vi "Update Available Channels.vi"(8 "error in (no error)":errorcluster) -> (0 "error out":errorcluster)   [LabVIEW 2016]
uses:
  <vilib>/TagLibrary/Create Tag (String).vi
  <vilib>/TagLibrary/Write (String).vi
  <vilib>/TagLibrary/Tag Library.lvlib
  <resource>/objmgr/daqmx.rc
  <vilib>/TagLibrary/Close Tag (Single).vi
panel:
  out "System Tag":string
  out "JSON string":string
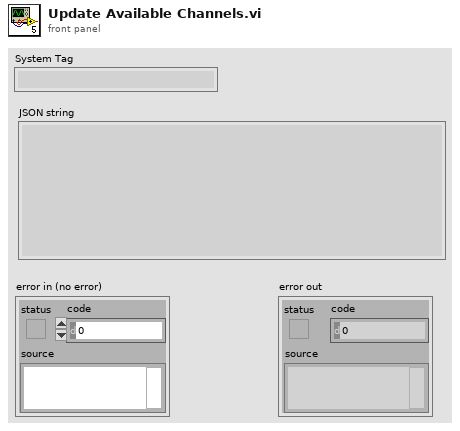
[diagram p1: front panel]
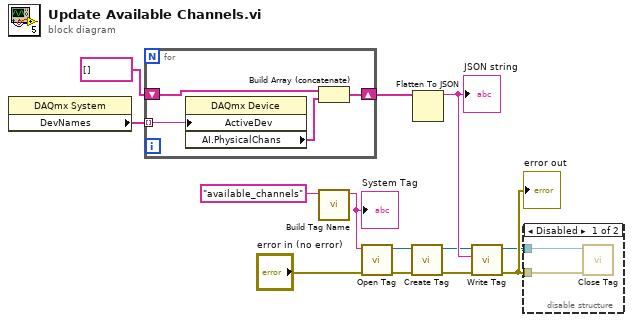
[diagram p0: block diagram]
diagram:
  n1 = property class="DAQmx System"() -> ("DevNames"=w10:tag[])  [unwired: 2 in, 2 out]
  n2 = for {
    tunnel: w10 -> [w17] mode=indexing
    shift-right: [w15] -> w1
    shift-left: string[] [] -> [w16]
    n3 = property class="DAQmx Device"("ActiveDev"=w17) -> ("AI.PhysicalChans"=w14:tag[])  [unwired: 2 in, 2 out]
    n4 = Build Array (concatenate)(w16, w14) -> (w15:string[])
  }
  n5 = call "Build Tag Name.vi"("Tag"="available_channels") -> ("System Tag"=w6:string)  [unwired: 10 in]
  "System Tag" <- w6
  n6 = call <vilib>:"Open Tag.vi"("error in (no error)"="error in (no error)", "tag path"=w6) -> ("error out"=w8:errorcluster, "tag reference out"=w7:refnum<k21>)  [unwired: 8 in]
  n7 = call-poly <vilib>:"Create Tag.vi"("error in (no error)"=w8, "tag reference in"=w7) -> ("error out"=w4:errorcluster, "tag reference out"=w5:refnum<k21>)  [unwired: 8 in]
  n8 = Flatten To JSON(anything=w1) -> (JSON string=w11:string)  [unwired: 2 in, 1 out]
  "JSON string" <- w11
  n9 = call-poly <vilib>:"Write Tag.vi"("error in (no error)"=w4, "string"=w11, "tag reference in"=w5) -> ("error out"=w13:errorcluster, "tag reference out"=w12:refnum<k21>)  [unwired: 7 in]
  "error out" <- w13
  n10 = disable-structure shown="Disabled" {
    disable-tunnel: w13 -> [w19 _]
    disable-tunnel: w12 -> [w18 _]
    frame Disabled {
      n11 = call-poly <vilib>:"Close Tag.vi"("error in (no error)"=w19, "tag reference"=w18) -> ()  [unwired: 9 in, 1 out]
    }
    frame Enabled {
    }
  }
